vi "main-top-level-example.vi"() -> ()   [LabVIEW 2024]
uses:
  controls/digital-output-cluster.ctl
  controls/thermocouple-input-cluster.ctl
  controls/analog-input-cluster.ctl
  controls/adam-5000-serial-settings.ctl
  controls/adam-5000-cmd-response.ctl
  controls/state-enum.ctl
  sub-vi/csv-file-logging/filepath-selection.ctl
  controls/adam-5000-all-chassis-data.ctl
  controls/adam-5000-all-module-datas.ctl
  controls/digitial-input-cluster.ctl
  controls/analog-output-cluster.ctl
  controls/adam-5000-chassis-cmd-ack.ctl
  controls/adam-5000-chassis-module-types.ctl
  controls/adam-5000-DO-user-input.ctl
  controls/adam-5000-status-indicator-references.ctl
panel:
  out "Hz":dbl format="%_3g"
  in  "Sample Rate (Hz)":dbl=1.0 min=0.0001 max=4.0 format="%#_4g"
  out "Logged Data String":string
  in  "CSV Data Headings":string="time (s),T1,T2,T3,T4,T5,T6,T7,T8,T9,T10,T11,T12,P1,P2,P3,P4"
  out "log-elapsed time":dbl format="%.2f"
  out "log start time":u32
  out "File Open":bool
  out "Log Filepath":path
  in  "Log Filepath Selection":T1={"Log Filepath Source"=enum."Application Relative (Auto)", "Log File Path (Manual)"=path "C:/Users/iwheard/Documents/0000-labview/adam5000-generic-controller/data", "Log File Folder Name"="data", "log file name"="log", "Include Date in Filename"=TRUE, "Include Time in Filename"=TRUE}
  out "Logging Active":bool
  out "Error Detected":bool
  in  "Reset":bool
  out "ADAM Connected":bool
  in  "Stop ADAM":bool
  in  "Start Logging":bool
  out "Program State":T2
  in  "Start ADAM":bool
  out "cmd-response":T4
  out "Status Indicators":T5
  in  "Debug Mode":bool
  out "1.Thermocouple Inputs (degC)":T6
  in  "5:Digital Outputs":T7
  in  "4:Digital Outputs":T7
  out "0:Analog Inputs":T8
  out "3:Thermocouple Inputs (degC)":T6
  in  "Chassis Settings":T9={"VISA resource name"="COM8", "baud rate (19200)"=19200, "Chassis ID"=1}
  out "Loop Time (mS)":u32
  out "Loop Counter":i32
  out "error":errorcluster
  in  "exit":bool
  # "ADAM 5000 Controller"
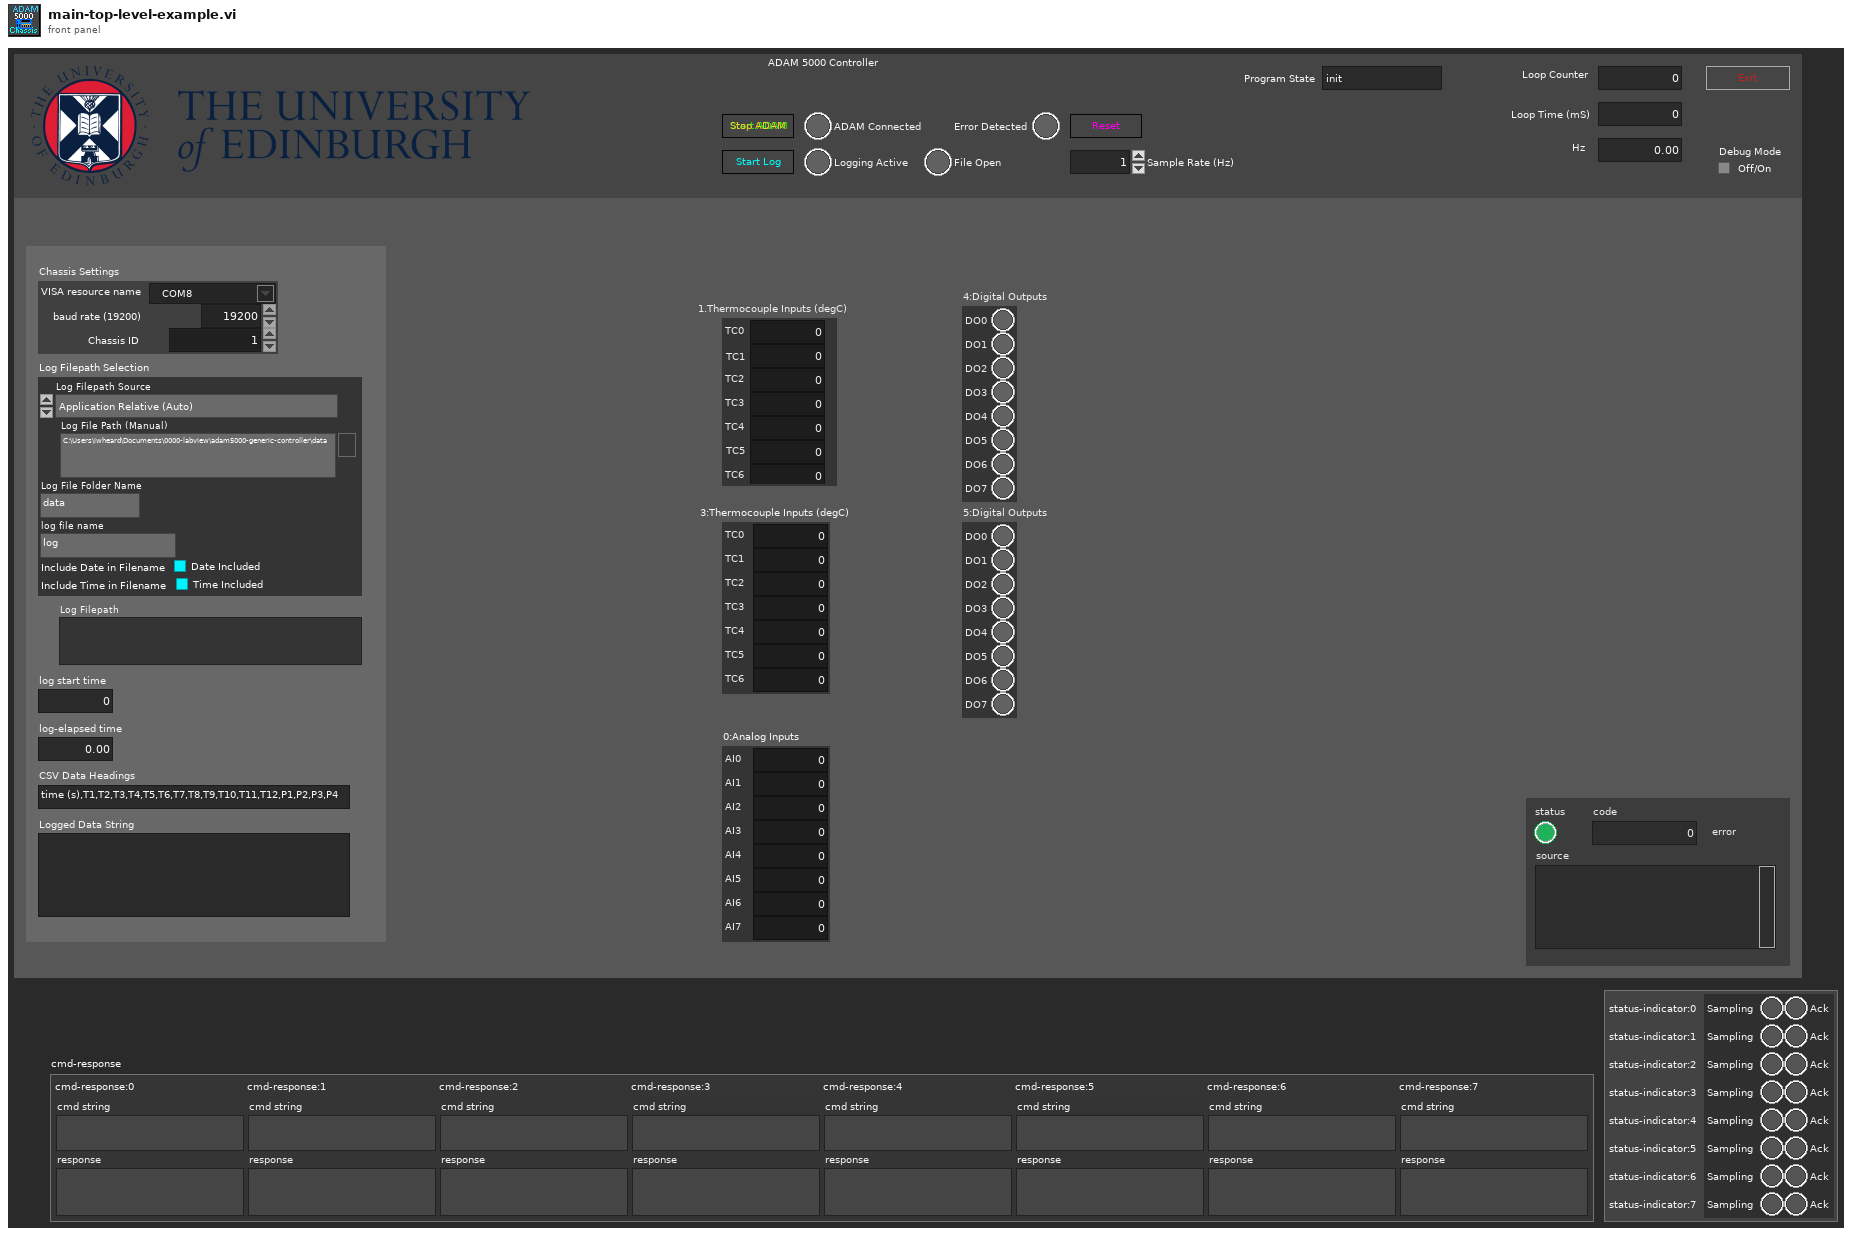
[diagram p1: front panel]
types:
  T1 = typedef "filepath-selection.ctl" = cluster{"Log Filepath Source":enum16{"Application Relative (Auto)", "VI Relative (Auto)", "Complete Path (Manual)"}, "Log File Path (Manual)":path, "Log File Folder Name":string, "log file name":string, "Include Date in Filename":bool, "Include Time in Filename":bool}
  T2 = typedef "state-enum.ctl" = enum16{"init", "wait", "manual", "start", "run", "reset", "stop", "exit"}
  T3 = typedef "adam-5000-cmd-response.ctl" = cluster{"cmd string":string, "response":string}
  T4 = cluster{"cmd-response:0":T3, "cmd-response:1":T3, "cmd-response:2":T3, "cmd-response:3":T3, "cmd-response:4":T3, "cmd-response:5":T3, "cmd-response:6":T3, "cmd-response:7":T3}
  T5 = cluster{"status-indicator:0":cluster{"Sampling":bool, "Ack":bool}, "status-indicator:1":cluster{"Sampling":bool, "Ack":bool}, "status-indicator:2":cluster{"Sampling":bool, "Ack":bool}, "status-indicator:3":cluster{"Sampling":bool, "Ack":bool}, "status-indicator:4":cluster{"Sampling":bool, "Ack":bool}, "status-indicator:5":cluster{"Sampling":bool, "Ack":bool}, "status-indicator:6":cluster{"Sampling":bool, "Ack":bool}, "status-indicator:7":cluster{"Sampling":bool, "Ack":bool}}
  T6 = typedef "thermocouple-input-cluster.ctl" = cluster{"TC0":dbl, "TC1":dbl, "TC2":dbl, "TC3":dbl, "TC4":dbl, "TC5":dbl, "TC6":dbl}
  T7 = typedef "digital-output-cluster.ctl" = cluster{"DO0":bool, "DO1":bool, "DO2":bool, "DO3":bool, "DO4":bool, "DO5":bool, "DO6":bool, "DO7":bool}
  T8 = typedef "analog-input-cluster.ctl" = cluster{"AI0":dbl, "AI1":dbl, "AI2":dbl, "AI3":dbl, "AI4":dbl, "AI5":dbl, "AI6":dbl, "AI7":dbl}
  T9 = typedef "adam-5000-serial-settings.ctl" = cluster{"VISA resource name":refnum<visa-resource-name>, "baud rate (19200)":u32, "Chassis ID":u8}
  T10 = enum16{"Digital Output", "Digital Input", "Analog Output", "Analog Input", "Thermocouple", "Power Relay", "empty"}
  T11 = typedef "adam-5000-chassis-module-types.ctl" = cluster{"Slot 0: Module Type":enum16{"Digital Output", "Digital Input", "Analog Output", "Analog Input", "Thermocouple", "Power Relay", "empty"}, "Slot 1: Module Type":enum16{"Digital Output", "Digital Input", "Analog Output", "Analog Input", "Thermocouple", "Power Relay", "empty"}, "Slot 2: Module Type":enum16{"Digital Output", "Digital Input", "Analog Output", "Analog Input", "Thermocouple", "Power Relay", "empty"}, "Slot 3: Module Type":enum16{"Digital Output", "Digital Input", "Analog Output", "Analog Input", "Thermocouple", "Power Relay", "empty"}, "Slot 4: Module Type":enum16{"Digital Output", "Digital Input", "Analog Output", "Analog Input", "Thermocouple", "Power Relay", "empty"}, "Slot 5: Module Type":enum16{"Digital Output", "Digital Input", "Analog Output", "Analog Input", "Thermocouple", "Power Relay", "empty"}, "Slot 6: Module Type":enum16{"Digital Output", "Digital Input", "Analog Output", "Analog Input", "Thermocouple", "Power Relay", "empty"}, "Slot 7: Module Type":enum16{"Digital Output", "Digital Input", "Analog Output", "Analog Input", "Thermocouple", "Power Relay", "empty"}}
  T12 = typedef "adam-5000-chassis-cmd-ack.ctl" = cluster{"cmd-response:0":T3, "cmd-response:1":T3, "cmd-response:2":T3, "cmd-response:3":T3, "cmd-response:4":T3, "cmd-response:5":T3, "cmd-response:6":T3, "cmd-response:7":T3}
  T13 = typedef "adam-5000-all-chassis-data.ctl" = cluster{"slot:0":T14, "slot:1":T14, "slot:2":T14, "slot:3":T14, "slot:4":T14, "slot:5":T14, "slot:6":T14, "slot:7":T14}
  T14 = typedef "adam-5000-all-module-datas.ctl" = cluster{"Digital Outputs":T7, "Digital Inputs":T15, "Analog Outputs":T16, "Analog Inputs":T8, "Thermocouple Inputs (degC)":T6}
  T15 = typedef "digitial-input-cluster.ctl" = cluster{"DI0":bool, "DI1":bool, "DI2":bool, "DI3":bool, "DI4":bool, "DI5":bool, "DI6":bool, "DI7":bool}
  T16 = typedef "analog-output-cluster.ctl" = cluster{"AO0":dbl, "AO1":dbl, "AO2":dbl, "AO3":dbl}
  T17 = enum8{"Enabled", "Disabled", "Disabled and Grayed Out"}
  T18 = typedef "adam-5000-status-indicator-references.ctl" = cluster{"status-indicator:0":refnum<vi>, "status-indicator:1":refnum<vi>, "status-indicator:2":refnum<vi>, "status-indicator:3":refnum<vi>, "status-indicator:4":refnum<vi>, "status-indicator:5":refnum<vi>, "status-indicator:6":refnum<vi>, "status-indicator:7":refnum<vi>}
  T19 = typedef "adam-5000-DO-user-input.ctl" = cluster{"0:Digital Outputs":T7, "1:Digital Outputs":T7, "2:Digital Outputs":T7, "3:Digital Outputs":T7, "4:Digital Outputs":T7, "5:Digital Outputs":T7, "6:Digital Outputs":T7, "7:Digital Outputs":T7}
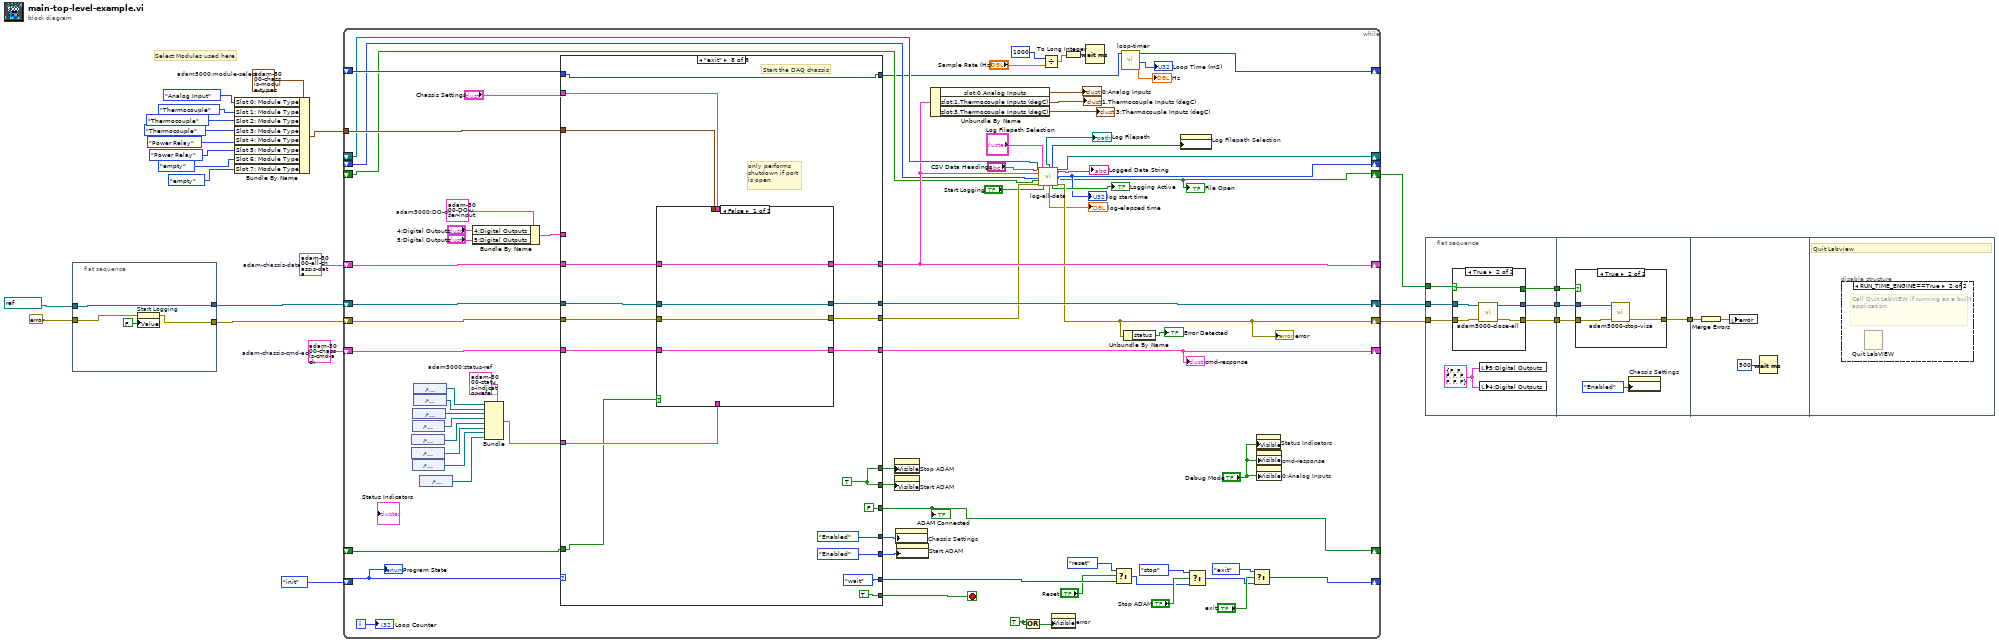
[diagram p0: block diagram]
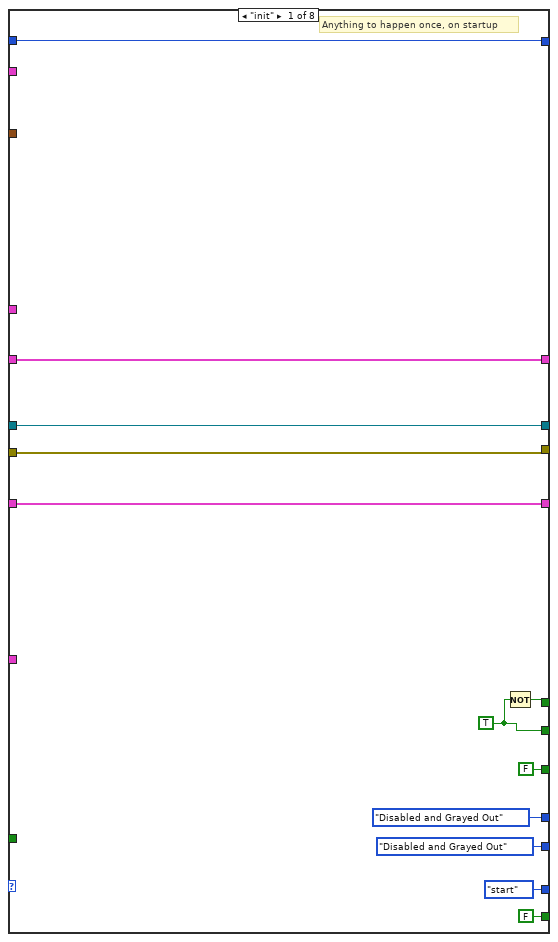
[diagram p5: hidden frame]
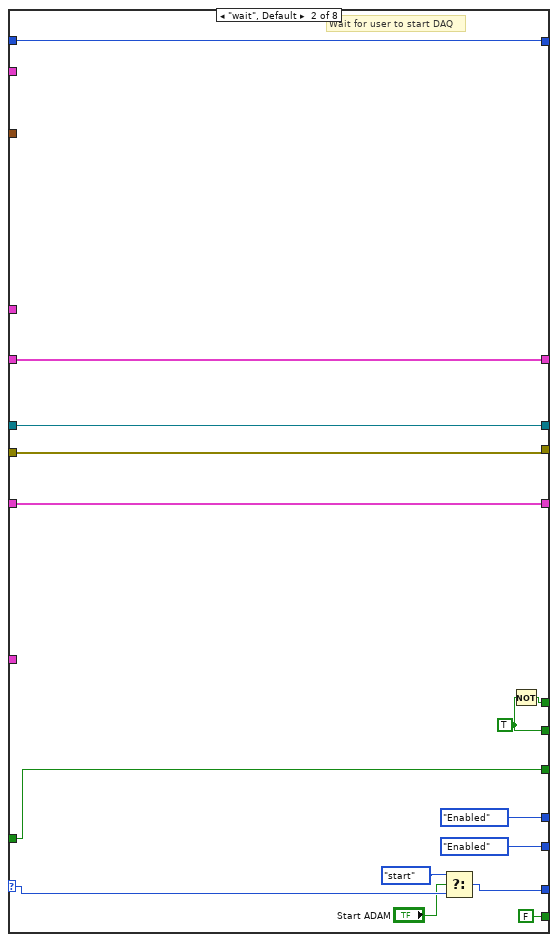
[diagram p6: hidden frame]
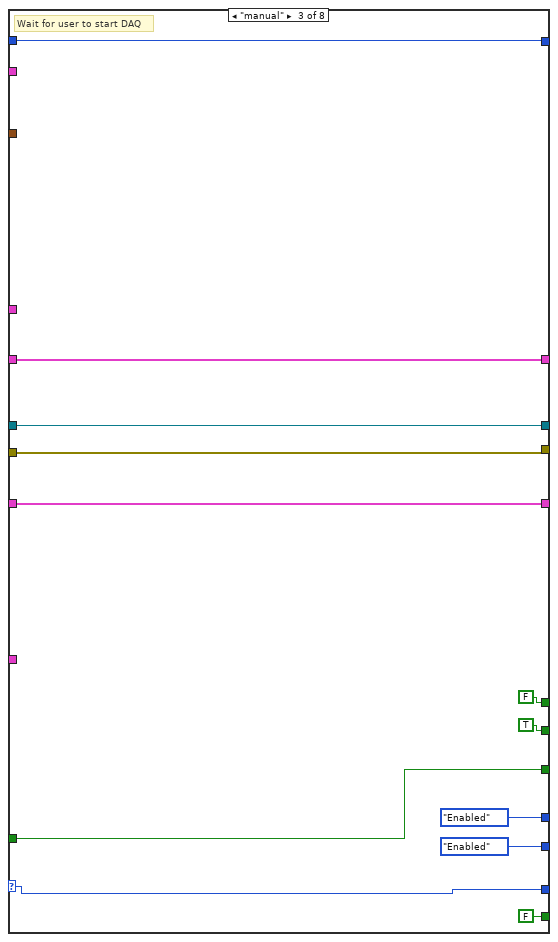
[diagram p7: hidden frame]
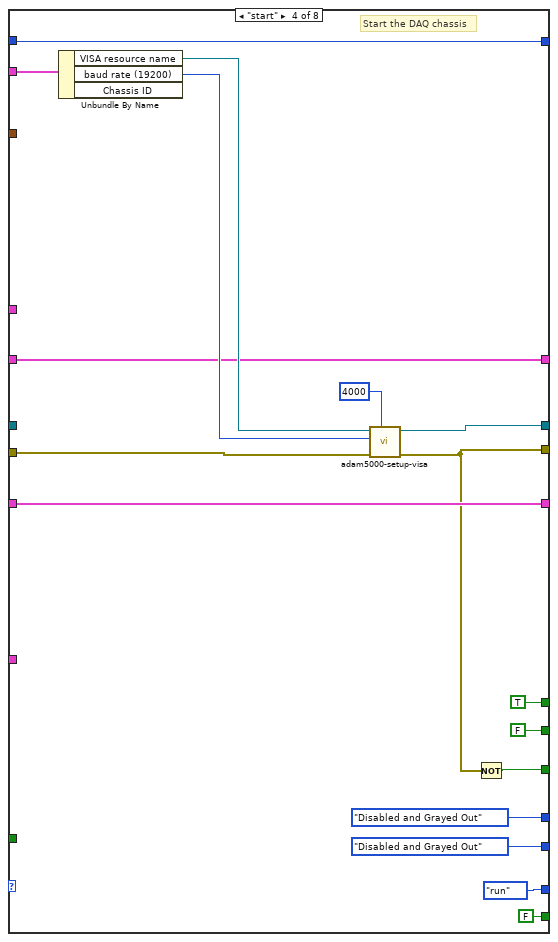
[diagram p8: hidden frame]
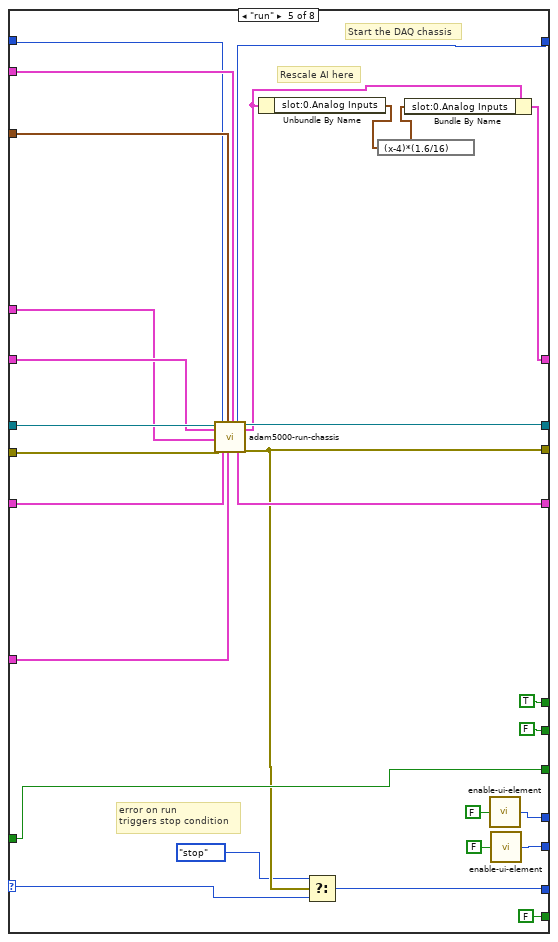
[diagram p9: hidden frame]
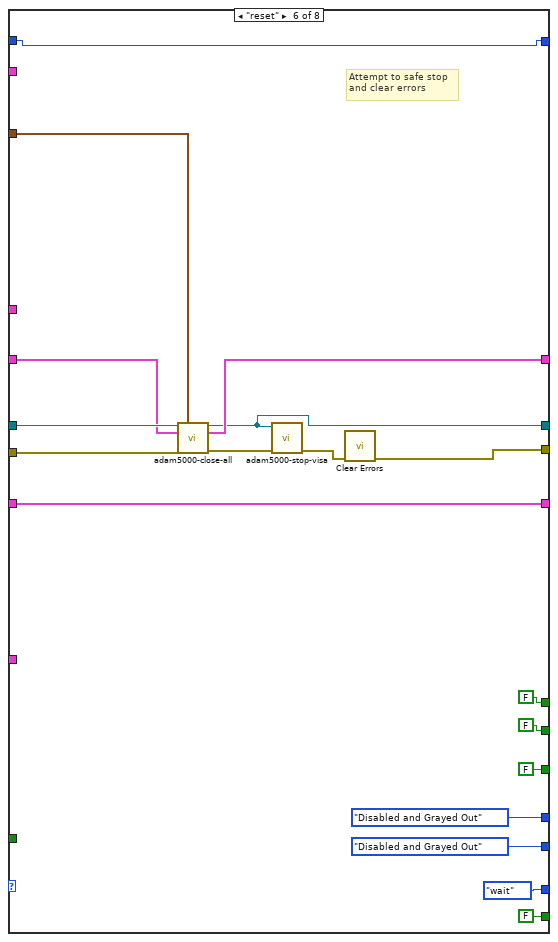
[diagram p10: hidden frame]
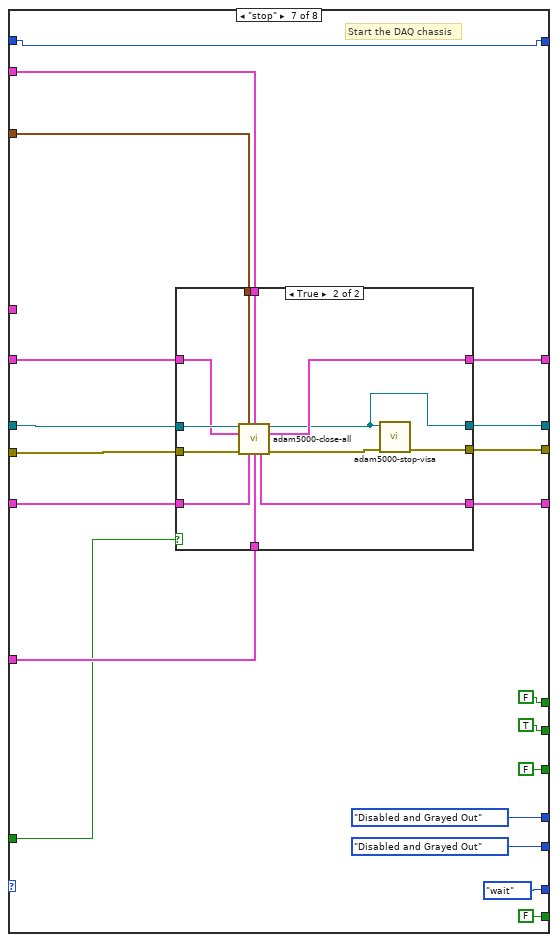
[diagram p11: hidden frame]
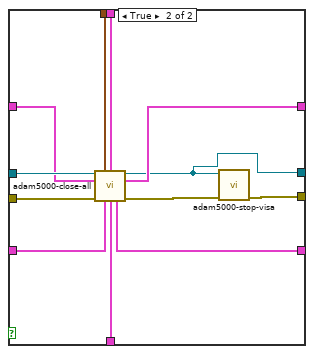
[diagram p13: hidden frame]
diagram:
  w16 = T11 {"Slot 0: Module Type"=enum."Digital Output", "Slot 1: Module Type"=enum."Digital Output", "Slot 2: Module Type"=enum."Digital Output", "Slot 3: Module Type"=enum."Digital Output", "Slot 4: Module Type"=enum."Digital Output", "Slot 5: Module Type"=enum."Digital Output", "Slot 6: Module Type"=enum."Digital Output", "Slot 7: Module Type"=enum."Digital Output"}  # adam5000:module-select
  w21 = T12 {"cmd-response:0"={"cmd string"="", "response"=""}, "cmd-response:1"={"cmd string"="", "response"=""}, "cmd-response:2"={"cmd string"="", "response"=""}, "cmd-response:3"={"cmd string"="", "response"=""}, "cmd-response:4"={"cmd string"="", "response"=""}, "cmd-response:5"={"cmd string"="", "response"=""}, "cmd-response:6"={"cmd string"="", "response"=""}, "cmd-response:7"={"cmd string"="", "response"=""}}  # adam-chassis-cmd-ack
  w22 = T13 {"slot:0"={"Digital Outputs"={"DO0"=FALSE, "DO1"=FALSE, "DO2"=FALSE, "DO3"=FALSE, "DO4"=FALSE, "DO5"=FALSE, "DO6"=FALSE, "DO7"=FALSE}, "Digital Inputs"={"DI0"=FALSE, "DI1"=FALSE, "DI2"=FALSE, "DI3"=FALSE, "DI4"=FALSE, "DI5"=FALSE, "DI6"=FALSE, "DI7"=FALSE}, "Analog Outputs"={"AO0"=0.0, "AO1"=0.0, "AO2"=0.0, "AO3"=0.0}, "Analog Inputs"={"AI0"=0.0, "AI1"=0.0, "AI2"=0.0, "AI3"=0.0, "AI4"=0.0, "AI5"=0.0, "AI6"=0.0, "AI7"=0.0}, "Thermocouple Inputs (degC)"={"TC0"=0.0, "TC1"=0.0, "TC2"=0.0, "TC3"=0.0, "TC4"=0.0, "TC5"=0.0, "TC6"=0.0}}, "slot:1"={"Digital Outputs"={"DO0"=FALSE, "DO1"=FALSE, "DO2"=FALSE, "DO3"=FALSE, "DO4"=FALSE, "DO5"=FALSE, "DO6"=FALSE, "DO7"=FALSE}, "Digital Inputs"={"DI0"=FALSE, "DI1"=FALSE, "DI2"=FALSE, "DI3"=FALSE, "DI4"=FALSE, "DI5"=FALSE, "DI6"=FALSE, "DI7"=FALSE}, "Analog Outputs"={"AO0"=0.0, "AO1"=0.0, "AO2"=0.0, "AO3"=0.0}, "Analog Inputs"={"AI0"=0.0, "AI1"=0.0, "AI2"=0.0, "AI3"=0.0, "AI4"=0.0, "AI5"=0.0, "AI6"=0.0, "AI7"=0.0}, "Thermocouple Inputs (degC)"={"TC0"=0.0, "TC1"=0.0, "TC2"=0.0, "TC3"=0.0, "TC4"=0.0, "TC5"=0.0, "TC6"=0.0}}, "slot:2"={"Digital Outputs"={"DO0"=FALSE, "DO1"=FALSE, "DO2"=FALSE, "DO3"=FALSE, "DO4"=FALSE, "DO5"=FALSE, "DO6"=FALSE, "DO7"=FALSE}, "Digital Inputs"={"DI0"=FALSE, "DI1"=FALSE, "DI2"=FALSE, "DI3"=FALSE, "DI4"=FALSE, "DI5"=FALSE, "DI6"=FALSE, "DI7"=FALSE}, "Analog Outputs"={"AO0"=0.0, "AO1"=0.0, "AO2"=0.0, "AO3"=0.0}, "Analog Inputs"={"AI0"=0.0, "AI1"=0.0, "AI2"=0.0, "AI3"=0.0, "AI4"=0.0, "AI5"=0.0, "AI6"=0.0, "AI7"=0.0}, "Thermocouple Inputs (degC)"={"TC0"=0.0, "TC1"=0.0, "TC2"=0.0, "TC3"=0.0, "TC4"=0.0, "TC5"=0.0, "TC6"=0.0}}, "slot:3"={"Digital Outputs"={"DO0"=FALSE, "DO1"=FALSE, "DO2"=FALSE, "DO3"=FALSE, "DO4"=FALSE, "DO5"=FALSE, "DO6"=FALSE, "DO7"=FALSE}, "Digital Inputs"={"DI0"=FALSE, "DI1"=FALSE, "DI2"=FALSE, "DI3"=FALSE, "DI4"=FALSE, "DI5"=FALSE, "DI6"=FALSE, "DI7"=FALSE}, "Analog Outputs"={"AO0"=0.0, "AO1"=0.0, "AO2"=0.0, "AO3"=0.0}, "Analog Inputs"={"AI0"=0.0, "AI1"=0.0, "AI2"=0.0, "AI3"=0.0, "AI4"=0.0, "AI5"=0.0, "AI6"=0.0, "AI7"=0.0}, "Thermocouple Inputs (degC)"={"TC0"=0.0, "TC1"=0.0, "TC2"=0.0, "TC3"=0.0, "TC4"=0.0, "TC5"=0.0, "TC6"=0.0}}, "slot:4"={"Digital Outputs"={"DO0"=FALSE, "DO1"=FALSE, "DO2"=FALSE, "DO3"=FALSE, "DO4"=FALSE, "DO5"=FALSE, "DO6"=FALSE, "DO7"=FALSE}, "Digital Inputs"={"DI0"=FALSE, "DI1"=FALSE, "DI2"=FALSE, "DI3"=FALSE, "DI4"=FALSE, "DI5"=FALSE, "DI6"=FALSE, "DI7"=FALSE}, "Analog Outputs"={"AO0"=0.0, "AO1"=0.0, "AO2"=0.0, "AO3"=0.0}, "Analog Inputs"={"AI0"=0.0, "AI1"=0.0, "AI2"=0.0, "AI3"=0.0, "AI4"=0.0, "AI5"=0.0, "AI6"=0.0, "AI7"=0.0}, "Thermocouple Inputs (degC)"={"TC0"=0.0, "TC1"=0.0, "TC2"=0.0, "TC3"=0.0, "TC4"=0.0, "TC5"=0.0, "TC6"=0.0}}, "slot:5"={"Digital Outputs"={"DO0"=FALSE, "DO1"=FALSE, "DO2"=FALSE, "DO3"=FALSE, "DO4"=FALSE, "DO5"=FALSE, "DO6"=FALSE, "DO7"=FALSE}, "Digital Inputs"={"DI0"=FALSE, "DI1"=FALSE, "DI2"=FALSE, "DI3"=FALSE, "DI4"=FALSE, "DI5"=FALSE, "DI6"=FALSE, "DI7"=FALSE}, "Analog Outputs"={"AO0"=0.0, "AO1"=0.0, "AO2"=0.0, "AO3"=0.0}, "Analog Inputs"={"AI0"=0.0, "AI1"=0.0, "AI2"=0.0, "AI3"=0.0, "AI4"=0.0, "AI5"=0.0, "AI6"=0.0, "AI7"=0.0}, "Thermocouple Inputs (degC)"={"TC0"=0.0, "TC1"=0.0, "TC2"=0.0, "TC3"=0.0, "TC4"=0.0, "TC5"=0.0, "TC6"=0.0}}, "slot:6"={"Digital Outputs"={"DO0"=FALSE, "DO1"=FALSE, "DO2"=FALSE, "DO3"=FALSE, "DO4"=FALSE, "DO5"=FALSE, "DO6"=FALSE, "DO7"=FALSE}, "Digital Inputs"={"DI0"=FALSE, "DI1"=FALSE, "DI2"=FALSE, "DI3"=FALSE, "DI4"=FALSE, "DI5"=FALSE, "DI6"=FALSE, "DI7"=FALSE}, "Analog Outputs"={"AO0"=0.0, "AO1"=0.0, "AO2"=0.0, "AO3"=0.0}, "Analog Inputs"={"AI0"=0.0, "AI1"=0.0, "AI2"=0.0, "AI3"=0.0, "AI4"=0.0, "AI5"=0.0, "AI6"=0.0, "AI7"=0.0}, "Thermocouple Inputs (degC)"={"TC0"=0.0, "TC1"=0.0, "TC2"=0.0, "TC3"=0.0, "TC4"=0.0, "TC5"=0.0, "TC6"=0.0}}, "slot:7"={"Digital Outputs"={"DO0"=FALSE, "DO1"=FALSE, "DO2"=FALSE, "DO3"=FALSE, "DO4"=FALSE, "DO5"=FALSE, "DO6"=FALSE, "DO7"=FALSE}, "Digital Inputs"={"DI0"=FALSE, "DI1"=FALSE, "DI2"=FALSE, "DI3"=FALSE, "DI4"=FALSE, "DI5"=FALSE, "DI6"=FALSE, "DI7"=FALSE}, "Analog Outputs"={"AO0"=0.0, "AO1"=0.0, "AO2"=0.0, "AO3"=0.0}, "Analog Inputs"={"AI0"=0.0, "AI1"=0.0, "AI2"=0.0, "AI3"=0.0, "AI4"=0.0, "AI5"=0.0, "AI6"=0.0, "AI7"=0.0}, "Thermocouple Inputs (degC)"={"TC0"=0.0, "TC1"=0.0, "TC2"=0.0, "TC3"=0.0, "TC4"=0.0, "TC5"=0.0, "TC6"=0.0}}}  # adam-chassis-data
  # "Select Modules used here"
  n1 = flat-sequence {
    tunnel: [w27] -> w5
    tunnel: refnum<visa-resource-name> "COM8" ("VISA Refnum out") -> [w27]
    tunnel: errorcluster {"status"=FALSE, "code"=0, "source"=""} ("error in") -> [w26]
    tunnel: [w25] -> w3
    frame #0 {
      n2 = property on="Start Logging" class="Bool (strict)"(error in=w26, "Value"=FALSE ("Start Logging")) -> (error out=w25:errorcluster)  [unwired: 1 in, 1 out]
    }
  }
  n3 = Bundle By Name(cluster=w16, "Slot 0: Module Type"=T10."Analog Input", "Slot 1: Module Type"=T10."Thermocouple", "Slot 2: Module Type"=T10."Thermocouple" ("Slot 1: Module Type"), "Slot 3: Module Type"=T10."Thermocouple" ("Slot 1: Module Type"), "Slot 4: Module Type"=T10."Power Relay" ("Slot 1: Module Type"), "Slot 5: Module Type"=T10."Power Relay" ("Slot 1: Module Type"), "Slot 6: Module Type"=T10."empty" ("Slot 1: Module Type"), "Slot 7: Module Type"=T10."empty" ("Slot 1: Module Type")) -> (w7:T11)
  n4 = while {
    shift-right: [w77] -> _
    shift-left: state-enum."init" ("state-enum") -> [w57]
    shift-right: [w37] -> _
    shift-left: _ -> [w82]
    shift-right: [w66] -> w20
    shift-left: w5 -> [w85]
    shift-right: [w43] -> w19
    shift-left: w3 -> [w84]
    shift-right: [w46] -> _
    shift-left: w22 -> [w81]
    shift-right: [w59] -> _
    shift-left: w21 -> [w79]
    shift-right: [w64] -> _
    shift-left: _ -> [w65]
    tunnel: w7 -> [w58]
    shift-right: [w29] -> w2
    shift-left: _ -> [w44]
    shift-right: [w30] -> _
    shift-left: _ -> [w45]
    shift-right: [w50] -> _
    shift-left: _ -> [w53]
    i -> [w102]
    stop <- w67 stop-if-true
    w89 = T18 {"status-indicator:0"=refnum, "status-indicator:1"=refnum, "status-indicator:2"=refnum, "status-indicator:3"=refnum, "status-indicator:4"=refnum, "status-indicator:5"=refnum, "status-indicator:6"=refnum, "status-indicator:7"=refnum}  # adam5000:status-ref
    w92 = T19 {"0:Digital Outputs"={"DO0"=FALSE, "DO1"=FALSE, "DO2"=FALSE, "DO3"=FALSE, "DO4"=FALSE, "DO5"=FALSE, "DO6"=FALSE, "DO7"=FALSE}, "1:Digital Outputs"={"DO0"=FALSE, "DO1"=FALSE, "DO2"=FALSE, "DO3"=FALSE, "DO4"=FALSE, "DO5"=FALSE, "DO6"=FALSE, "DO7"=FALSE}, "2:Digital Outputs"={"DO0"=FALSE, "DO1"=FALSE, "DO2"=FALSE, "DO3"=FALSE, "DO4"=FALSE, "DO5"=FALSE, "DO6"=FALSE, "DO7"=FALSE}, "3:Digital Outputs"={"DO0"=FALSE, "DO1"=FALSE, "DO2"=FALSE, "DO3"=FALSE, "DO4"=FALSE, "DO5"=FALSE, "DO6"=FALSE, "DO7"=FALSE}, "4:Digital Outputs"={"DO0"=FALSE, "DO1"=FALSE, "DO2"=FALSE, "DO3"=FALSE, "DO4"=FALSE, "DO5"=FALSE, "DO6"=FALSE, "DO7"=FALSE}, "5:Digital Outputs"={"DO0"=FALSE, "DO1"=FALSE, "DO2"=FALSE, "DO3"=FALSE, "DO4"=FALSE, "DO5"=FALSE, "DO6"=FALSE, "DO7"=FALSE}, "6:Digital Outputs"={"DO0"=FALSE, "DO1"=FALSE, "DO2"=FALSE, "DO3"=FALSE, "DO4"=FALSE, "DO5"=FALSE, "DO6"=FALSE, "DO7"=FALSE}, "7:Digital Outputs"={"DO0"=FALSE, "DO1"=FALSE, "DO2"=FALSE, "DO3"=FALSE, "DO4"=FALSE, "DO5"=FALSE, "DO6"=FALSE, "DO7"=FALSE}}  # adam5000:DO-ch
    w68 = TRUE ("Debug Mode")
    n5 = control-ref of="status-indicator:4"() -> (w96:refnum<vi>)
    n6 = control-ref of="status-indicator:5"() -> (w95:refnum<vi>)
    n7 = control-ref of="status-indicator:3"() -> (w97:refnum<vi>)
    n8 = control-ref of="status-indicator:6"() -> (w94:refnum<vi>)
    n9 = control-ref of="status-indicator:2"() -> (w98:refnum<vi>)
    n10 = control-ref of="status-indicator:0"() -> (w100:refnum<vi>)
    n11 = control-ref of="status-indicator:1"() -> (w99:refnum<vi>)
    n12 = control-ref of="status-indicator:7"() -> (w93:refnum<vi>)
    n13 = Bundle By Name(cluster=w92, "4:Digital Outputs"="4:Digital Outputs", "5:Digital Outputs"="5:Digital Outputs") -> (w80:T19)
    n14 = Bundle(cluster=w89, "status-indicator:0"=w100, "status-indicator:1"=w99, "status-indicator:2"=w98, "status-indicator:3"=w97, "status-indicator:4"=w96, "status-indicator:5"=w95, "status-indicator:6"=w94, "status-indicator:7"=w93) -> (w78:T18)
    n15 = case shown="\"exit\"" w57 {
      selector: w57 -> [_ w127 w137 _ w171 _ _ _]
      tunnel: [state-enum."start" ("state-enum") w128 w137 state-enum."run" ("state-enum") w172 state-enum."wait" ("state-enum") state-enum."wait" ("state-enum") state-enum."wait" ("state-enum")] -> w62
      tunnel: [T17."Disabled and Grayed Out" ("Disabled") T17."Enabled" ("Disabled") T17."Enabled" ("Disabled") T17."Disabled and Grayed Out" ("Disabled") w161 T17."Disabled and Grayed Out" ("Disabled") T17."Disabled and Grayed Out" ("Disabled") T17."Enabled" ("Disabled")] -> w87
      tunnel: [T17."Disabled and Grayed Out" ("Disabled") T17."Enabled" ("Disabled") T17."Enabled" ("Disabled") T17."Disabled and Grayed Out" ("Disabled") w159 T17."Disabled and Grayed Out" ("Disabled") T17."Disabled and Grayed Out" ("Disabled") T17."Enabled" ("Disabled")] -> w86
      tunnel: w85 -> [w111 w124 w139 _ w186 w195 w221 w256]
      tunnel: [w111 w124 w139 w156 w184 w189 w211 w244] -> w66
      tunnel: w84 -> [w110 w123 w138 w155 w185 w194 w220 w255]
      tunnel: [w110 w123 w138 w145 w170 w198 w210 w245] -> w42
      tunnel: "Chassis Settings" -> [_ _ _ w154 w183 _ w218 w253]
      tunnel: w58 -> [_ _ _ _ w182 w191 w219 w254]
      tunnel: w82 -> [w109 w121 w136 w149 w181 w200 w212 w247]
      tunnel: [w109 w121 w136 w149 w180 w200 w212 w247] -> w38
      tunnel: w81 -> [w108 w120 w135 w148 w179 w193 w217 w252]
      tunnel: w80 -> [_ _ _ _ w178 _ _ _]
      tunnel: w79 -> [w107 w119 w134 w147 w177 w199 w215 w250]
      tunnel: w78 -> [_ _ _ _ w176 _ w214 w249]
      tunnel: [w107 w119 w134 w147 w175 w199 w213 w248] -> w59
      tunnel: [w108 w120 w135 w148 w165 w192 w216 w251] -> w46
      tunnel: [FALSE FALSE FALSE FALSE FALSE FALSE FALSE TRUE] -> w67
      tunnel: [FALSE w117 w132 w144 w173 FALSE FALSE FALSE] -> w64
      tunnel: w65 -> [_ w117 w132 _ w173 _ w207 w242]
      tunnel: [w104 w115 TRUE ("Visible") FALSE ("Visible") FALSE ("Visible") FALSE ("Visible") TRUE ("Visible") w241] -> w56
      tunnel: [w103 w116 FALSE ("Visible") TRUE ("Visible") TRUE ("Visible") FALSE ("Visible") FALSE ("Visible") w241] -> w55
      frame "init" {
        w104 = TRUE ("Visible")
        # "Anything to happen once, on startup"
        n16 = Not(x=w104) -> (.not. x?=w103:bool)
      }
      frame "wait", Default {
        w115 = TRUE ("Visible")
        # "Wait for user to start DAQ"
        n17 = Select(t=state-enum."start" ("state-enum"), s="Start ADAM", f=w127) -> (s? t:f=w128:T2)
        n18 = Not(x=w115) -> (.not. x?=w116:bool)
      }
      frame "manual" {
        # "Wait for user to start DAQ"
      }
      frame "start" {
        # "Start the DAQ chassis"
        n19 = Unbundle By Name(w154) -> ("VISA resource name"=w153:refnum<visa-resource-name>, "baud rate (19200)"=w152:u32)  [unwired: 1 out]
        n20 = call "adam5000-setup-visa.vi"("timeout (10sec)"=u32 4000, "error in"=w155, "baud rate (19200)"=w152, "VISA Refnum in"=w153) -> ("error out"=w145:errorcluster, "VISA Refnum out"=w156:refnum<visa-resource-name>)  [unwired: 6 in]
        n21 = Not(x=w145) -> (.not. x?=w144:bool)
      }
      frame "run" {
        # "Rescale AI here"
        # "error on run\ntriggers stop condition"
        # "Start the DAQ chassis"
        n22 = call "adam5000-run-chassis.vi"("VISA Refnum In"=w186, "adam-chassis-all-data-in"=w179, "adam-chassis-all-DO-in"=w178, "error in"=w185, "loop-time-in"=w181, "adam-chassis-cmd-response-in"=w177, "adam-chassis-module-select-in"=w182, "adam5000:status-ref-in"=w176, "Chassis Settings"=w183) -> ("loop-time-out"=w180:u32, "adam-chassis-cmd-response-out"=w175:T12, "VISA Refnum Out"=w184:refnum<visa-resource-name>, "adam-chassis-all-data-out"=w166:T13, "error out"=w170:errorcluster)  [unwired: 5 in, 1 out]
        n23 = Unbundle By Name(w166) -> ("slot:0.Analog Inputs"=w164:T8)
        n24 = Select(t=state-enum."stop", s=w170, f=w171) -> (s? t:f=w172:T2)
        n25 = expression code="(x-4)*(1.6/16)"(w164) -> (w163:T8)
        n26 = Bundle By Name(cluster=w166, "slot:0.Analog Inputs"=w163) -> (w165:T13)
        n27 = call "enable-ui-element.vi"("Enable UI Element"=FALSE) -> ("UI Element State"=w161:T17)  [unwired: 8 in]
        n28 = call "enable-ui-element.vi"("Enable UI Element"=FALSE) -> ("UI Element State"=w159:T17)  [unwired: 8 in]
      }
      frame "reset" {
        # "Attempt to safe stop\nand clear errors"
        n29 = call "adam5000-close-all.vi"("VISA Refnum in"=w195, "adam5000:module-type-select"=w191, "adam5000:all-data-in"=w193, "error in (no error)"=w194) -> ("VISA Refnum out"=w189:refnum<visa-resource-name>, "adam5000:all-data-out"=w192:T13, "error out"=w196:errorcluster)  [unwired: 8 in, 1 out]
        n30 = call "adam5000-stop-visa.vi"("error in (no error)"=w196, "VISA resource in"=w189) -> ("error out"=w190:errorcluster)  [unwired: 9 in]
        n31 = call <vilib>:"Clear Errors.vi"("error in (no error)"=w190) -> ("error out"=w198:errorcluster)  [unwired: 5 in, 1 out]
      }
      frame "stop" {
        # "Start the DAQ chassis"
        n32 = case shown="True" w207 {
          tunnel: w221 -> [w226 w240]
          tunnel: w220 -> [w225 w239]
          tunnel: w219 -> [_ w238]
          tunnel: w218 -> [_ w237]
          tunnel: w217 -> [w228 w236]
          tunnel: [w228 w235] -> w216
          tunnel: w215 -> [w227 w234]
          tunnel: w214 -> [_ w233]
          tunnel: [w227 w232] -> w213
          tunnel: [w226 w231] -> w211
          tunnel: [w225 w229] -> w210
          frame False {
          }
          frame True {
            n33 = call "adam5000-close-all.vi"("VISA Refnum in"=w240, "adam5000:module-type-select"=w238, "Chassis Settings in"=w237, "adam5000:all-data-in"=w236, "error in (no error)"=w239, "adam-chassis-cmd-ack"=w234, "adam5000:status-ref"=w233) -> ("VISA Refnum out"=w231:refnum<visa-resource-name>, "adam5000:all-data-out"=w235:T13, "adam-chassis-cmd-response-out"=w232:T12, "error out"=w230:errorcluster)  [unwired: 5 in]
            n34 = call "adam5000-stop-visa.vi"("error in (no error)"=w230, "VISA resource in"=w231) -> ("error out"=w229:errorcluster)  [unwired: 9 in]
          }
        }
      }
      frame "exit" {
        w241 = TRUE ("Visible")
        # "only performs\nshutdown if port\nis open"
        # "Start the DAQ chassis"
        n35 = case shown="False" w242 {
          tunnel: w256 -> [w262 w275]
          tunnel: w255 -> [w261 w274]
          tunnel: w254 -> [_ w273]
          tunnel: w253 -> [_ w272]
          tunnel: w252 -> [w263 w271]
          tunnel: [w263 w270] -> w251
          tunnel: w250 -> [w260 w269]
          tunnel: w249 -> [_ w268]
          tunnel: [w260 w267] -> w248
          tunnel: [w261 w265] -> w245
          tunnel: [w262 w264] -> w244
          frame False {
          }
          frame True {
            n36 = call "adam5000-close-all.vi"("VISA Refnum in"=w275, "adam5000:module-type-select"=w273, "Chassis Settings in"=w272, "adam5000:all-data-in"=w271, "error in (no error)"=w274, "adam-chassis-cmd-ack"=w269, "adam5000:status-ref"=w268) -> ("VISA Refnum out"=w264:refnum<visa-resource-name>, "adam5000:all-data-out"=w270:T13, "adam-chassis-cmd-response-out"=w267:T12, "error out"=w266:errorcluster)  [unwired: 5 in]
            n37 = call "adam5000-stop-visa.vi"("error in (no error)"=w266, "VISA resource in"=w264) -> ("error out"=w265:errorcluster)  [unwired: 9 in]
          }
        }
      }
    }
    "cmd-response" <- w59
    "ADAM Connected" <- w64
    n38 = property on="Stop ADAM" class="Bool"("Visible"=w55) -> ()  [unwired: 2 in, 2 out]
    n39 = property on="Start ADAM" class="Bool"("Visible"=w56) -> ()  [unwired: 2 in, 2 out]
    n40 = property on="Chassis Settings" class="Clust (strict)"("DisabledEnum"=w87) -> ()  [unwired: 2 in, 2 out]
    n41 = property on="Start ADAM" class="Bool"("DisabledEnum"=w86) -> ()  [unwired: 2 in, 2 out]
    n42 = Unbundle By Name(w46) -> ("slot:0.Analog Inputs"=→"0:Analog Inputs":T8, "slot:1.Thermocouple Inputs (degC)"=→"1.Thermocouple Inputs (degC)":T6, "slot:3.Thermocouple Inputs (degC)"=→"3:Thermocouple Inputs (degC)":T6)
    n43 = Or(x=w68, y=w68) -> (x .or. y?=w101:bool)
    n44 = call "log-all-data.vi"("log-file-byte-stream"=w53, "CSV Data Headings"="CSV Data Headings", "adam5000:all-data-in"=w46, "log-start-time(mS)"=w45, "file open?"=w44, "error in (no error)"=w42, "Log Filepath Selection"="Log Filepath Selection", "Start Logging"="Start Logging") -> ("appended path for log file"=→"Log Filepath":path, "log-elapsed time"=→"log-elapsed time":dbl, "log-filepath-enable-state"=w49:T17, "Start Logging"=→"Logging Active":bool, "log-file-bytestream"=w50:refnum<file>, "Logged Data String"=→"Logged Data String":string, "log-start-time(mS)"=w30:u32, "file open?"=w29:bool, "error out"=w43:errorcluster)  [unwired: 3 in]
    "error" <- w43
    "File Open" <- w29
    "log start time" <- w30
    n45 = Divide(x=u32 1000 ("milliseconds to wait"), y="Sample Rate (Hz)") -> (x/y=w32:dbl)
    n46 = property on="error" class="Clust (strict)"("Visible"=w101) -> ()  [unwired: 2 in, 2 out]
    n47 = To Long Integer(number=w32) -> (32bit integer=w31:i32)
    n48 = Wait (ms)(milliseconds to wait=w31) -> ()  [unwired: 1 out]
    n49 = Select(t=state-enum."reset", s="Reset", f=w62) -> (s? t:f=w61:T2)
    n50 = call "loop-timer.vi"("loop-time-in"=w38) -> ("Loop Time (mS)"=→"Loop Time (mS)":u32, "loop-time-out"=w37:u32, "Hz"=→"Hz":dbl)  [unwired: 8 in]
    n51 = Unbundle By Name(w43) -> ("status"=→"Error Detected":bool)
    n52 = property on="Log Filepath Selection" class="Clust (strict)"("DisabledEnum"=w49) -> ()  [unwired: 2 in, 2 out]
    n53 = Select(t=state-enum."stop", s="Stop ADAM", f=w61) -> (s? t:f=w71:T2)
    n54 = Select(t=state-enum."exit", s="exit", f=w71) -> (s? t:f=w77:T2)
    n55 = property on="Status Indicators" class="Clust (strict)"("Visible"="Debug Mode") -> ()  [unwired: 2 in, 2 out]
    n56 = property on="cmd-response" class="Clust (strict)"("Visible"="Debug Mode") -> ()  [unwired: 2 in, 2 out]
    n57 = property on="0:Analog Inputs" class="Clust (strict)"("Visible"="Debug Mode") -> ()  [unwired: 2 in, 2 out]
    "Loop Counter" <- w102
    "Program State" <- w57
  }
  n58 = flat-sequence {
    tunnel: w20 -> [w282]
    tunnel: w19 -> [w281]
    tunnel: [w280] -> w18
    tunnel: [w279] -> w17
    tunnel: w2 -> [w277]
    tunnel: [w276] -> w1
    tunnel: [w295] -> w23
    tunnel: w18 -> [w294]
    tunnel: w17 -> [w293]
    tunnel: w1 -> [w291]
    tunnel: w23 -> [w301]
    frame #0 {
      w278 = T7 {"DO0"=FALSE, "DO1"=FALSE, "DO2"=FALSE, "DO3"=FALSE, "DO4"=FALSE, "DO5"=FALSE, "DO6"=FALSE, "DO7"=FALSE} ("5:Digital Outputs")
      n59 = case shown="True" w277 {
        selector: w277 -> [w283 w286]
        tunnel: w282 -> [w285 w290]
        tunnel: w281 -> [w284 w289]
        tunnel: [w284 w288] -> w280
        tunnel: [w285 w287] -> w279
        tunnel: [w283 w286] -> w276
        frame False {
        }
        frame True {
          n60 = call "adam5000-close-all.vi"("VISA Refnum in"=w290, "error in (no error)"=w289) -> ("VISA Refnum out"=w287:refnum<visa-resource-name>, "error out"=w288:errorcluster)  [unwired: 10 in, 2 out]
        }
      }
      n61 = local write "5:Digital Outputs"(w278) -> ()
      n62 = local write "4:Digital Outputs"(w278) -> ()
    }
    frame #1 {
      n63 = case shown="True" w291 {
        tunnel: [w296 w299] -> w295
        tunnel: w294 -> [w296 w298]
        tunnel: w293 -> [_ w297]
        frame False {
        }
        frame True {
          n64 = call "adam5000-stop-visa.vi"("error in (no error)"=w298, "VISA resource in"=w297) -> ("error out"=w299:errorcluster)  [unwired: 9 in]
        }
      }
      n65 = property on="Chassis Settings" class="Clust (strict)"("DisabledEnum"=T17."Enabled" ("Disabled")) -> ()  [unwired: 2 in, 2 out]
    }
    frame #2 {
      n66 = Merge Errors(w301) -> (w300:errorcluster)
      n67 = local write "error"(w300) -> ()
      n68 = Wait (ms)(milliseconds to wait=u32 500) -> ()  [unwired: 1 out]
    }
    frame #3 {
      # "Quit Labview"
      n69 = disable-structure "Conditional Disable Structure" shown="RUN_TIME_ENGINE==True" {
        frame condition #0 (active) {
        }
        frame condition #1 {
          # "Call Quit LabVIEW if running as a built application."
          n70 = Quit LabVIEW() -> ()  [unwired: 1 in]
        }
      }
    }
  }
